vi "Write Pressure Servo Valve 2 Setpoint.vi"(10 "Pressure Servo Valve 2 Setpoint":dbl[unit], 11 "IActuatorCylinder in":refnum<class "ILCControlledActuatorCylinder.lvclass">) -> (3 "IActuatorCylinder out":refnum<class "ILCControlledActuatorCylinder.lvclass">)   [LabVIEW 2015, in "ILCControlledActuatorCylinder.lvclass"]
uses:
  ILCControlledActuatorCylinder.lvclass
  ILCControlledActuatorCylinder.lvclass/ILCControlledActuatorCylinder.ctl
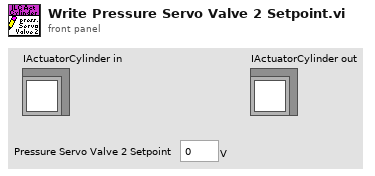
[diagram p1: front panel]
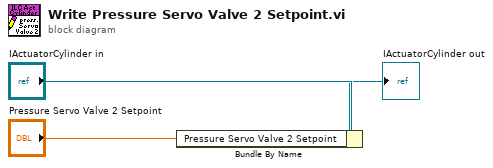
[diagram p0: block diagram]
diagram:
  n1 = Bundle By Name(cluster="IActuatorCylinder in", "Pressure Servo Valve 2 Setpoint"="Pressure Servo Valve 2 Setpoint") -> (→"IActuatorCylinder out":refnum<class "ILCControlledActuatorCylinder.lvclass">)
